vi "Loop.vi"(11 "TEMPLATE Event in":refnum<class "TEMPLATE Event.lvclass">) -> (3 "TEMPLATE Event out":refnum<class "TEMPLATE Event.lvclass">)   [LabVIEW 2021, in "_Template.lvlib" / "Templates.lvlib" / "TEMPLATE Event.lvlib" / "TEMPLATE Event.lvclass"]
uses:
  TEMPLATE Event.lvclass
  C:/Program Files/National Instruments/LabVIEW 2021/vi.lib/Nathan Davis/jettl/jettl/jettl/jettl.lvclass
  TEMPLATE Event.lvclass/TEMPLATE Event.ctl
  <vilib>/Nathan Davis/jettl/jettl/Event/Event.lvclass
  <vilib>/Nathan Davis/jettl/jettl/Msg Strategy/Msg Strategy.lvclass
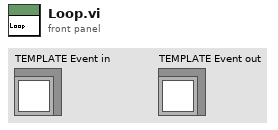
[diagram p1: front panel]
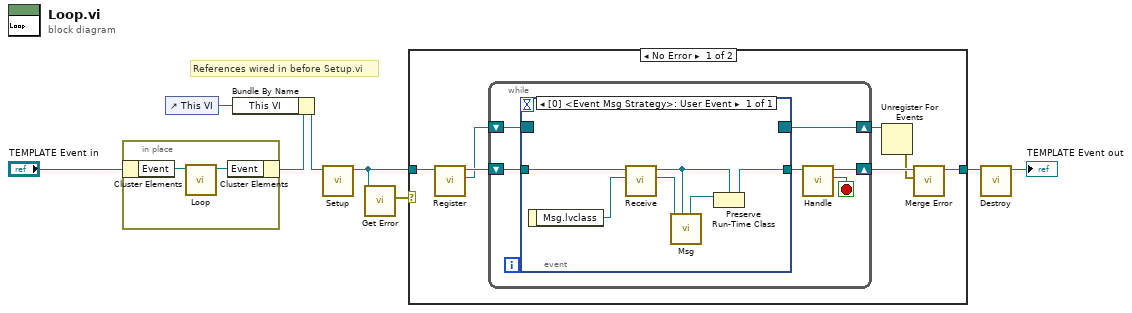
[diagram p0: block diagram]
diagram:
  # "References wired in before Setup.vi"
  n1 = in-place {
    n2 = in-place-cluster #1("TEMPLATE Event in") -> ("Event"=w10:refnum<class "Event.lvclass">)
    n3 = call-dynamic "Loop.vi"("Event in"=w10) -> ("Event out"=w9:refnum<class "Event.lvclass">)  [unwired: 10 in]
    n4 = in-place-cluster #1("Event"=w9) -> (w7:refnum<class "TEMPLATE Event.lvclass">)
  }
  n5 = control-ref of="This VI"() -> (w6:refnum<vi>)
  n6 = Bundle By Name(cluster=w7, "This VI"=w6) -> (w5:refnum<class "TEMPLATE Event.lvclass">)
  n7 = call-dynamic "Setup.vi"("TEMPLATE Event in"=w5) -> ("TEMPLATE Event out"=w3:refnum<class "TEMPLATE Event.lvclass">)  [unwired: 10 in]
  n8 = call-dynamic "Get Error.vi"("Template Event in"=w3) -> ("Error"=w4:errorcluster)  [unwired: 10 in]
  n9 = case shown="No Error" w4 {
    tunnel: w3 -> [w17 w30]
    tunnel: [w12 w30] -> w2
    frame No Error {
      n10 = call-dynamic "Register.vi"("Template Event in"=w17) -> ("Registration"=w14:refnum<event-registration>, "Template Event out"=w15:refnum<class "TEMPLATE Event.lvclass">)  [unwired: 9 in]
      n11 = while {
        shift-right: [w22] -> w16
        shift-left: w14 -> [w23]
        shift-right: [w19] -> w13
        shift-left: w15 -> [w21]
        stop <- w18 stop-if-true
        n12 = event shown="[0] <Event Msg Strategy>: User Event" {
          selector: w23 -> [_]
          dyn-events: [_] -> w22
          timeout: _ -> [_]
          tunnel: w21 -> [w27]
          tunnel: [w29] -> w20
          event User Event {
            n13 = event-data() -> ("Msg.lvclass"=w24:refnum<class "Msg Strategy.lvclass">)  [unwired: 1 in]
            n14 = call-dynamic "Receive.vi"("Msg Strategy in"=w24, "Template Event in"=w27) -> ("Msg Strategy out"=w25:refnum<class "Msg Strategy.lvclass">, "Template Event out"=w26:refnum<class "TEMPLATE Event.lvclass">)  [unwired: 8 in]
            n15 = call-dynamic "Msg.vi"("jettl in"=w26, "Msg Strategy in"=w25) -> ("jettl out"=w28:refnum<class "jettl.lvclass">)  [unwired: 9 in]
            n16 = Preserve Run-Time Class(object in=w28, 2:w26) -> (object out=w29:refnum<class "TEMPLATE Event.lvclass">)  [unwired: 1 in, 1 out]
          }
        }
        n17 = call-dynamic "Handle.vi"("Template Event in"=w20) -> ("Destroy?"=w18:bool, "Template Event out"=w19:refnum<class "TEMPLATE Event.lvclass">)  [unwired: 9 in]
      }
      n18 = Unregister For Events(event registration refnum=w16) -> (error out=w11:errorcluster)  [unwired: 1 in]
      n19 = call-dynamic "Merge Error.vi"("Error"=w11, "TEMPLATE Event in"=w13) -> ("TEMPLATE Event out"=w12:refnum<class "TEMPLATE Event.lvclass">)  [unwired: 9 in]
    }
    frame Error {
    }
  }
  n20 = call-dynamic "Destroy.vi"("Template Event in"=w2) -> ("Template Event out"=→"TEMPLATE Event out":refnum<class "TEMPLATE Event.lvclass">)  [unwired: 10 in]
